vi "saveLedgerSeeds.vi"(6 "error in (no error)":errorcluster, 8 "ExperimentDescriptors 2":T1, 9 "Recording":string, 10 "Date":string, 11 "dataRoot":path) -> (4 "error out":errorcluster)   [LabVIEW 2015]
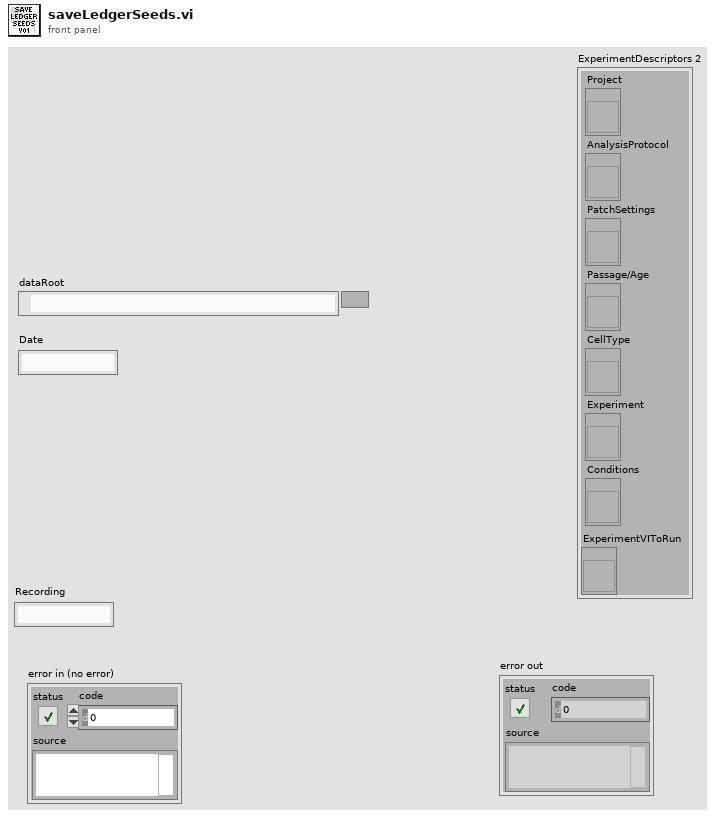
[diagram p1: front panel]
types:
  T1 = cluster{"Project":refnum<vi>, "AnalysisProtocol":refnum<vi>, "PatchSettings":refnum<vi>, "Passage/Age":refnum<vi>, "CellType":refnum<vi>, "Experiment":refnum<vi>, "Conditions":refnum<vi>, "ExperimentVIToRun":refnum<vi>}
  T2 = enum16{"open", "replace", "create", "open or create", "replace or create", "replace or create with confirmation"}
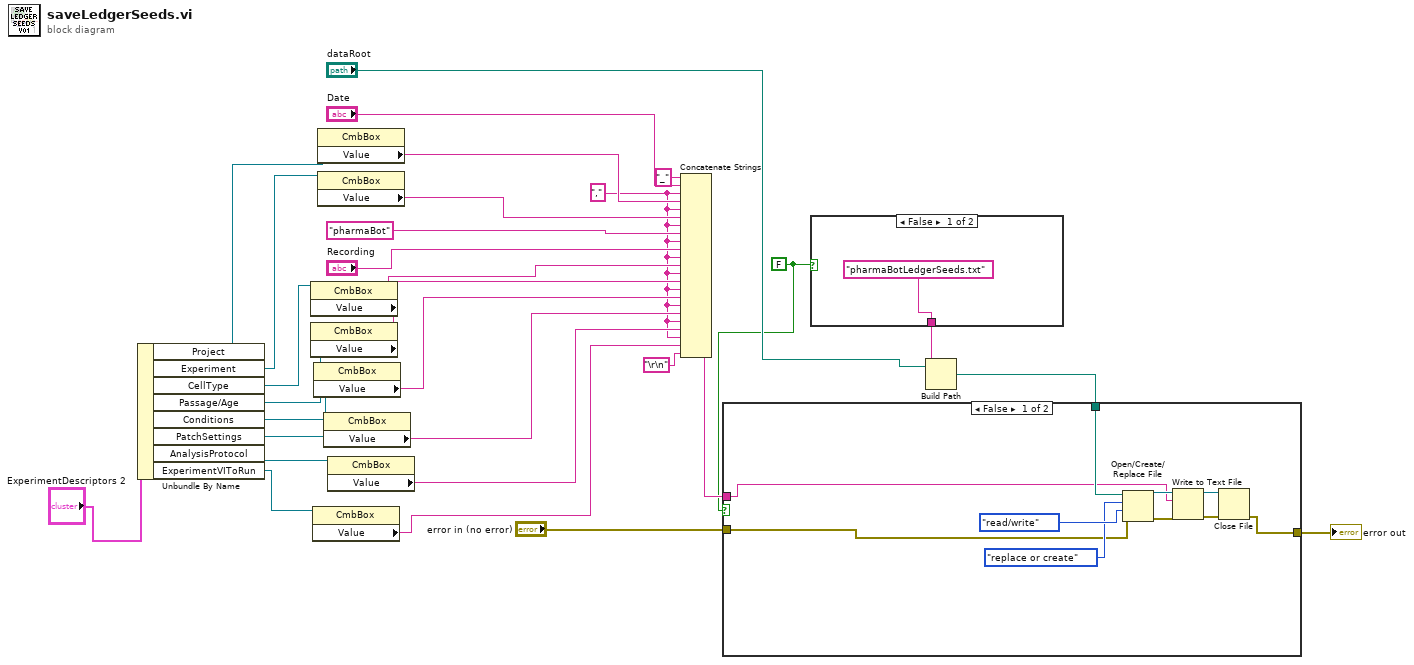
[diagram p0: block diagram]
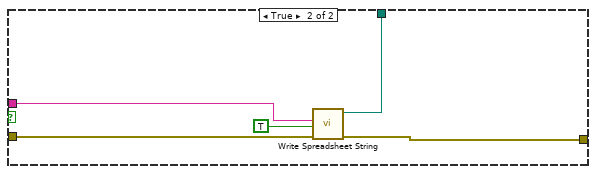
[diagram p2: hidden frame]
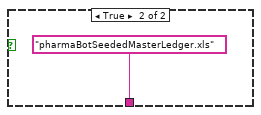
[diagram p3: hidden frame]
diagram:
  w2 = ","
  w7 = FALSE
  n1 = Unbundle By Name("ExperimentDescriptors 2") -> ("Project"=w24:refnum<vi>, "Experiment"=w22:refnum<vi>, "CellType"=w21:refnum<vi>, "Passage/Age"=w19:refnum<vi>, "Conditions"=w14:refnum<vi>, "PatchSettings"=w13:refnum<vi>, "AnalysisProtocol"=w12:refnum<vi>, "ExperimentVIToRun"=w4:refnum<vi>)
  n2 = property class="CmbBox"(reference=w21) -> ("Value"=w20:string)  [unwired: 1 in, 2 out]
  n3 = property class="CmbBox"(reference=w19) -> ("Value"=w18:string)  [unwired: 1 in, 2 out]
  n4 = property class="CmbBox"(reference=w4) -> ("Value"=w1:string)  [unwired: 1 in, 2 out]
  n5 = property class="CmbBox"(reference=w14) -> ("Value"=w11:string)  [unwired: 1 in, 2 out]
  n6 = property class="CmbBox"(reference=w24) -> ("Value"=w23:string)  [unwired: 1 in, 2 out]
  n7 = property class="CmbBox"(reference=w22) -> ("Value"=w15:string)  [unwired: 1 in, 2 out]
  n8 = property class="CmbBox"(reference=w13) -> ("Value"=w17:string)  [unwired: 1 in, 2 out]
  n9 = property class="CmbBox"(reference=w12) -> ("Value"=w16:string)  [unwired: 1 in, 2 out]
  n10 = Concatenate Strings("_" ("string"), "Date", w2, w23, w2, w15, w2, "pharmaBot", w2, "Recording", w2, w20, w2, w18, w2, w11, w2, w17, w2, w16, w2, w1, "\r\n") -> (w25:string)
  n11 = case shown="False" w7 {
    tunnel: ["pharmaBotLedgerSeeds.txt" "pharmaBotSeededMasterLedger.xls"] -> w9
    frame False {
    }
    frame True {
    }
  }
  n12 = Build Path(base path="dataRoot", name or relative path=w9) -> (appended path=w8:path)
  n13 = case shown="False" w7 {
    tunnel: [w34 w47] -> w27
    tunnel: "error in (no error)" -> [w33 w46]
    tunnel: w25 -> [w35 w44]
    tunnel: w8 -> [w36 w43]
    frame False {
      n14 = Open/Create/Replace File(file path (use dialog)=w36, error in=w33, operation (0:open)=T2."replace or create", access (0:read/write)=enum16{"read/write", "read-only", "write-only"}."read/write") -> (refnum out=w40:refnum<file>, error out=w41:errorcluster)  [unwired: 2 in, 1 out]
      n15 = Write to Text File(file (use dialog)=w40, text=w35, error in=w41) -> (refnum out=w38:refnum<file>, error out=w39:errorcluster)  [unwired: 1 in, 1 out]
      n16 = Close File(refnum=w38, error in=w39) -> (error out=w34:errorcluster)  [unwired: 1 out]
    }
    frame True {
      n17 = call <vilib>:"Write Spreadsheet String.vi"("error in"=w46, "append to file? (new file:F)"=TRUE, "spreadsheet string"=w44, "file path (dialog if empty)"=w43) -> ("error out"=w47:errorcluster)  [unwired: 6 in, 1 out]
    }
  }
  "error out" <- w27
